vi "Logical Sort.vi"(2 "Input Array":cluster{"date/time string":string, i32}[](array[cluster])) -> (7 "Sorted Array":cluster{"date/time string":string, i32}[](array[cluster]))   [LabVIEW 2020, in "TdmsFileViewer.lvlib"]
uses:
  TdmsFileViewer.lvlib
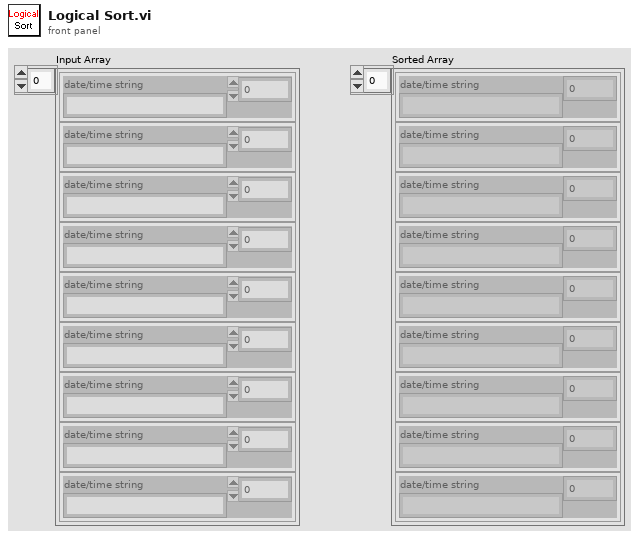
[diagram p1: front panel]
types:
  T1 = cluster{"split str":cluster{"str":string, "num":i32}[], "orig str":string, "index":i32}
  T2 = cluster{"split str":cluster{"str":string, "num":i32}[], "orig str":string, "index":i32}[]
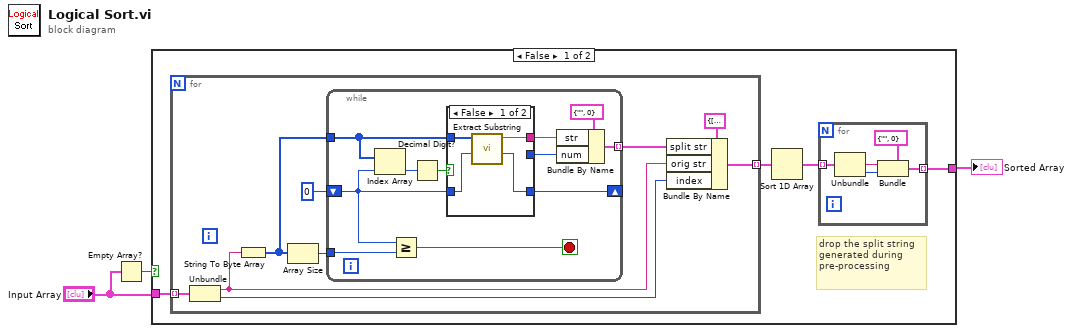
[diagram p0: block diagram]
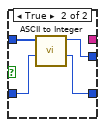
[diagram p2: hidden frame]
diagram:
  n1 = Empty Array?(array="Input Array") -> (empty?=w2:bool)
  n2 = case shown="False" w2 {
    tunnel: [w5 _] -> w1
    tunnel: "Input Array" -> [w7 _]
    frame False {
      # "drop the split string generated during\npre-processing"
      n3 = for {
        tunnel: w7 -> [w9] mode=indexing
        tunnel: [w10] -> w4 mode=indexing
        n4 = Unbundle(w9) -> ("date/time string"=w13:string, w12:i32)
        n5 = String To Byte Array(string=w13) -> (unsigned byte array=w15:u8[])
        n6 = Array Size(array=w15) -> (size(s)=w14:i32)
        n7 = while {
          shift-right: [w23] -> _
          shift-left: 0 ("size(s)") -> [w22]
          tunnel: w15 -> [w26]
          tunnel: w14 -> [w21]
          tunnel: [w17] -> w8 mode=indexing
          stop <- w19 stop-if-true
          n8 = Index Array(array=w26, index=w22) -> (element=w27:u8)
          n9 = Greater Or Equal?(x=w22, y=w21) -> (x >= y?=w19:bool)
          n10 = Decimal Digit?(1:w27) -> (0:w18:bool)
          n11 = case shown="False" w18 {
            tunnel: w26 -> [w29 w35]
            tunnel: [w28 _] -> w25
            tunnel: [_ w32] -> w24
            tunnel: w22 -> [w31 w34]
            tunnel: [w30 w33] -> w23
            frame False {
              n12 = call "Extract Substring.vi"("offset"=w31, "string byte array"=w29) -> ("new offset"=w30:i32, "sub string"=w28:string)  [unwired: 8 in]
            }
            frame True {
              n13 = call "ASCII to Integer.vi"("offset"=w34, "string byte array"=w35) -> ("new offset"=w33:i32, "value"=w32:i32)  [unwired: 8 in]
            }
          }
          n14 = Bundle By Name(cluster=cluster{"str":string, "num":i32} {"str"="", "num"=0}, "str"=w25, "num"=w24) -> (w17:cluster{"str":string, "num":i32})
        }
        n15 = Bundle By Name(cluster=T1 {"split str"=[], "orig str"="", "index"=0} ("Cluster"), "split str"=w8, "orig str"=w13, "index"=w12) -> (w10:T1)
      }
      n16 = Sort 1D Array(array=w4) -> (sorted array=w6:T2)
      n17 = for {
        tunnel: w6 -> [w40] mode=indexing
        tunnel: [w36] -> w5 mode=indexing
        n18 = Unbundle(w40) -> ("orig str"=w38:string, "index"=w37:i32)  [unwired: 1 out]
        n19 = Bundle(cluster=cluster{"date/time string":string, i32} {"date/time string"="", 0}, "date/time string"=w38, w37) -> (w36:cluster{"date/time string":string, i32})
      }
    }
    frame True {
    }
  }
  "Sorted Array" <- w1
